vi "Read SSH.vi"(8 "Error In":errorcluster, 11 "Session In":refnum<class "Session.lvclass">) -> (0 "Erorr Out":errorcluster, 2 "SSH":refnum<class "SSH.lvclass">, 3 "Session Out":refnum<class "Session.lvclass">)   [LabVIEW 2018, in "Toolkit.lvlib" / "Session.lvclass"]
uses:
  Session.lvclass
  SSH/SSH.lvclass
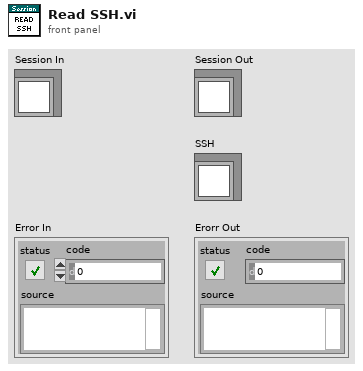
[diagram p1: front panel]
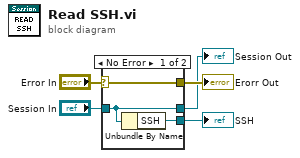
[diagram p0: block diagram]
diagram:
  n1 = case shown="No Error" "Error In" {
    selector: "Error In" -> [w8 w9]
    tunnel: [w8 w9] -> w4
    tunnel: "Session In" -> [w7 w10]
    tunnel: [w7 w10] -> w2
    tunnel: [w6 _] -> w1
    frame No Error {
      n2 = Unbundle By Name(w7) -> ("SSH"=w6:refnum<class "SSH.lvclass">)
    }
    frame Error {
    }
  }
  "Erorr Out" <- w4
  "Session Out" <- w2
  "SSH" <- w1
